vi "Write Data to file.vi"(8 "error in":errorcluster, 11 "Report Generator in":refnum<class "Report Generator.lvclass">) -> (0 "error out":errorcluster, 3 "Report Generator out":refnum<class "Report Generator.lvclass">)   [LabVIEW 2018, in "Report Generator.lvlib" / "Report Generator.lvclass"]
uses:
  Report Generator.lvclass
  Report Generator.lvclass/Report Generator.ctl
  <vilib>/Utility/file.llb/Write Delimited Spreadsheet (string).vi
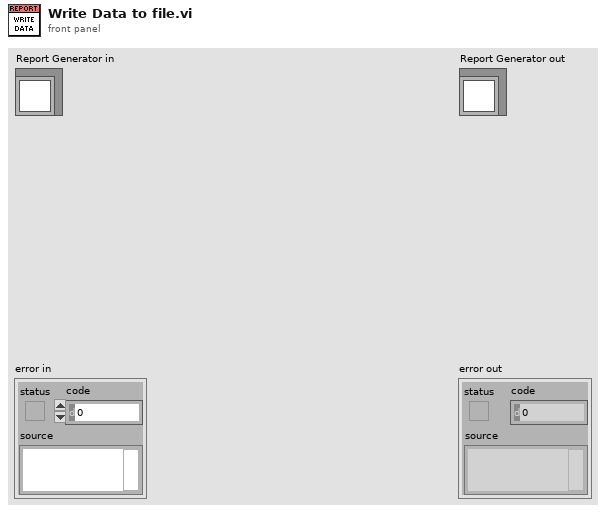
[diagram p1: front panel]
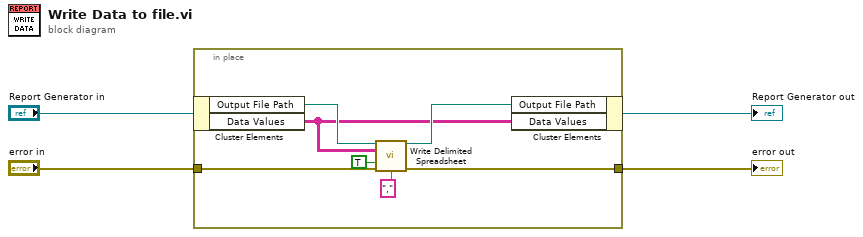
[diagram p0: block diagram]
diagram:
  n1 = in-place {
    in-place-border: [w8] -> w2
    in-place-border: "error in" -> [w6]
    n2 = in-place-cluster #1("Report Generator in") -> ("Output File Path"=w11:path, "Data Values"=w5:string[][])
    n3 = call-poly <vilib>:"Write Delimited Spreadsheet.vi"("file path (dialog if empty)"=w11, "2D data"=w5, "append to file? (new file:F)"=TRUE, "error in (no error)"=w6, "delimiter (\\t)"="," ("delimiter (\\t)")) -> ("new file path (Not A Path if cancelled)"=w10:path, "error out"=w8:errorcluster)  [unwired: 9 in]
    n4 = in-place-cluster #1("Output File Path"=w10, "Data Values"=w5) -> (→"Report Generator out":refnum<class "Report Generator.lvclass">)
  }
  "error out" <- w2
